vi "FPGA Input Write.vi"(8 "error in (no error)":errorcluster, 9 "Data":dbl, 10 "Input Register Info":T2, 11 "FPGA Session In":refnum<class "FPGA Interface Base.lvclass">) -> (0 "error out":errorcluster, 3 "FPGA Session Out":refnum<class "FPGA Interface Base.lvclass">)   [LabVIEW 2010, in "Sensor Simulation Custom Device.lvlib"]
uses:
  Sensor Simulation Custom Device.lvlib
  <userlib>/_FPGA Interface Advanced Tools/FPGA Interface Base/FPGA Interface Base.lvclass
  TypeDefs/InputChannelTypes.ctl
  <userlib>/_FPGA Interface Advanced Tools/FPGA Interface Base/FPGA Write By Name - U64.vi
  <userlib>/AES/RT/AES RT.lvlib
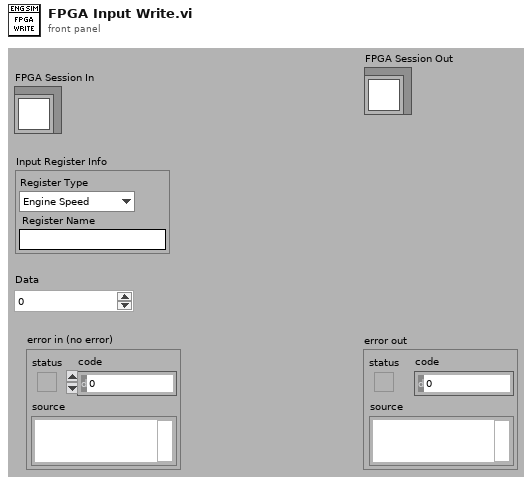
[diagram p1: front panel]
types:
  T1 = typedef "Sensor Simulation Custom Device.lvlib/InputChannelTypes.ctl" = enum16{"Engine Speed", "Offset"}
  T2 = cluster{"Register Type":T1, "Register Name":string}
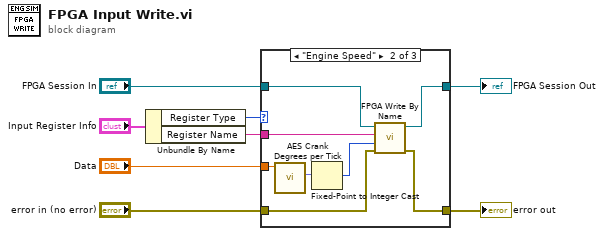
[diagram p0: block diagram]
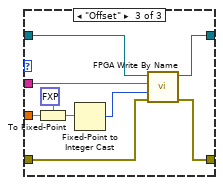
[diagram p3: hidden frame]
diagram:
  n1 = Unbundle By Name("Input Register Info") -> ("Register Type"=w7:T1, "Register Name"=w6:string)
  n2 = case shown="\"Engine Speed\"" w7 {
    tunnel: w6 -> [_ w14 w27]
    tunnel: "FPGA Session In" -> [w10 w15 w26]
    tunnel: [w10 w12 w25] -> w4
    tunnel: "Data" -> [_ w18 w22]
    tunnel: "error in (no error)" -> [w9 w13 w24]
    tunnel: [w9 w11 w23] -> w1
    frame Default {
    }
    frame "Engine Speed" {
      n3 = call <userlib>:"AES Crank Degrees per Tick.vi"("RPM"=w18) -> ("degrees per tick"=w17:fxp<+/-,47,-4>)  [unwired: 9 in, 1 out]
      n4 = Fixed-Point to Integer Cast(1:w17) -> (0:w16:i64)
      n5 = call-poly <userlib>:"FPGA Write By Name.vi"("error in (no error)"=w13, "Value"=w16, "Control"=w14, "FPGA Session In"=w15) -> ("error out"=w11:errorcluster, "FPGA Session Out"=w12:refnum<class "FPGA Interface Base.lvclass">)  [unwired: 6 in]
    }
    frame "Offset" {
      n6 = To Fixed-Point(fixed-point type=fxp<+/-,61,10> 0.0 ("FullyCustomTeeth.Cams.Cam1.Offset"), number=w22) -> (fixed-point=w20:fxp<+/-,61,10>)
      n7 = Fixed-Point to Integer Cast(1:w20) -> (0:w19:i64)
      n8 = call-poly <userlib>:"FPGA Write By Name.vi"("error in (no error)"=w24, "Value"=w19, "Control"=w27, "FPGA Session In"=w26) -> ("error out"=w23:errorcluster, "FPGA Session Out"=w25:refnum<class "FPGA Interface Base.lvclass">)  [unwired: 6 in]
    }
  }
  "FPGA Session Out" <- w4
  "error out" <- w1
